vi "Get All Property.vi"(8 "error in":errorcluster, 11 "Item Ref in":refnum<data-value>) -> (0 "error out":errorcluster, 3 "Properties out":refnum<class "Property.lvclass">[](array[class]))   [LabVIEW 2024, in "Config File Parser.lvlib" / "Property.lvclass"]
uses:
  Property.lvclass
  Property.lvclass/Property.ctl
  Item/Item.lvclass
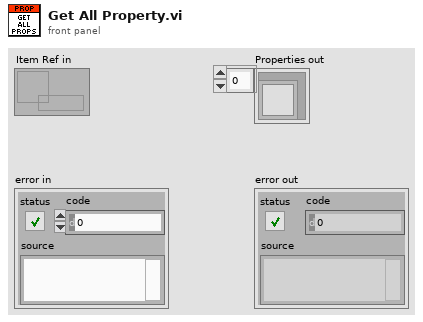
[diagram p1: front panel]
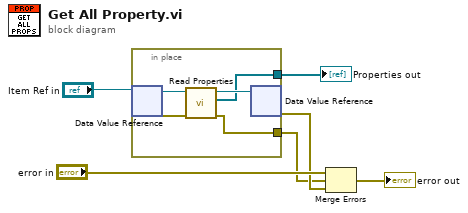
[diagram p0: block diagram]
diagram:
  n1 = in-place "In Place Element Structure" {
    in-place-border: [w10] -> w3
    in-place-border: [w7] -> w1
    n2 = in-place-dvr #1("Item Ref in") -> (w9:refnum<class "Item.lvclass">, w11:errorcluster)
    n3 = call-dynamic "Read Properties.vi"("error in (no error)"=w11, "Item in"=w9) -> ("error out"=w10:errorcluster, "Properties"=w7:refnum<class "Property.lvclass">[], "Item out"=w8:refnum<class "Item.lvclass">)  [unwired: 7 in]
    n4 = in-place-dvr #1(w8) -> (w5:errorcluster)  [unwired: 1 out]
  }
  "Properties out" <- w1
  n5 = Merge Errors("error in", w3, w5) -> (→"error out":errorcluster)
